vi "Complex Ratio.vi"(9 "Results":dbl[][](array[numeric]), 10 "Lock-in denominator":T1 items=["Lock-in #1", "Lock-in #2", "Lock-in #3", "Lock-in #4"], 11 "Lock-in numerator":T1 items=["Lock-in #1", "Lock-in #2", "Lock-in #3", "Lock-in #4"]) -> (3 "Array":dbl[](array[numeric]))   [LabVIEW 2013]
uses:
  Lockin.ctl
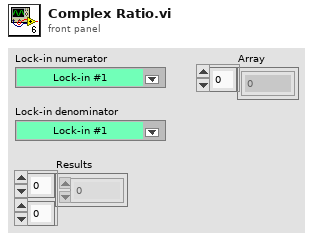
[diagram p1: front panel]
types:
  T1 = typedef "Lockin.ctl" = u16
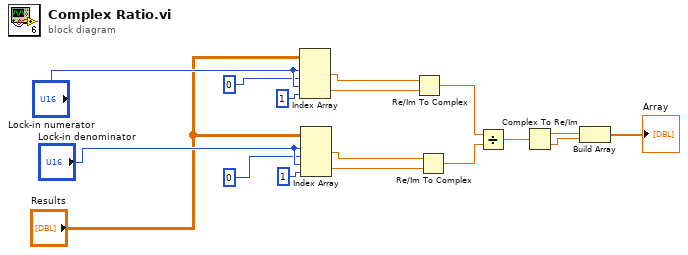
[diagram p0: block diagram]
diagram:
  n1 = Index Array(array="Results", index (row) #1="Lock-in numerator", index (col) #1=0 ("disabled index (col)"), index (row) #2="Lock-in numerator", index (col) #2=1 ("disabled index (col)")) -> (element #1=w8:dbl, element #2=w9:dbl)
  n2 = Index Array(array="Results", index (row) #1="Lock-in denominator", index (col) #1=0 ("disabled index (col)"), index (row) #2="Lock-in denominator", index (col) #2=1 ("disabled index (col)")) -> (element #1=w10:dbl, element #2=w11:dbl)
  n3 = Re/Im To Complex(1:w9, 2:w8) -> (0:w3:cdb)
  n4 = Re/Im To Complex(1:w11, 2:w10) -> (0:w2:cdb)
  n5 = Divide(x=w3, y=w2) -> (x/y=w1:cdb)
  n6 = Complex To Re/Im(x + iy=w1) -> (x=w15:dbl, y=w16:dbl)
  n7 = Build Array(w15, w16) -> (→"Array":dbl[])
